vi "Longueur d'onde.vi"(11 "T thermistances":dbl[](array[numeric])) -> (3 "Wavelenght":dbl format="%#_13g")   [LabVIEW 2018]
uses:
  <vilib>/Analysis/baseanly.llb/Mean (DBL).vi
  <vilib>/Analysis/NI_AALBase.lvlib
  <vilib>/gmath/NI_Gmath.lvlib
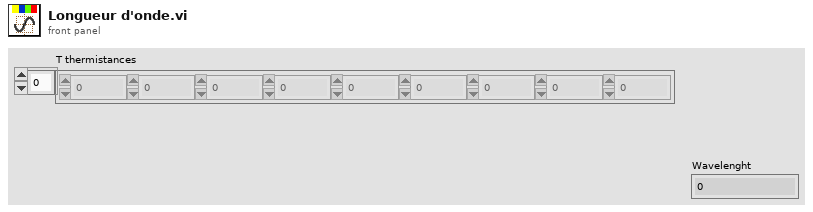
[diagram p1: front panel]
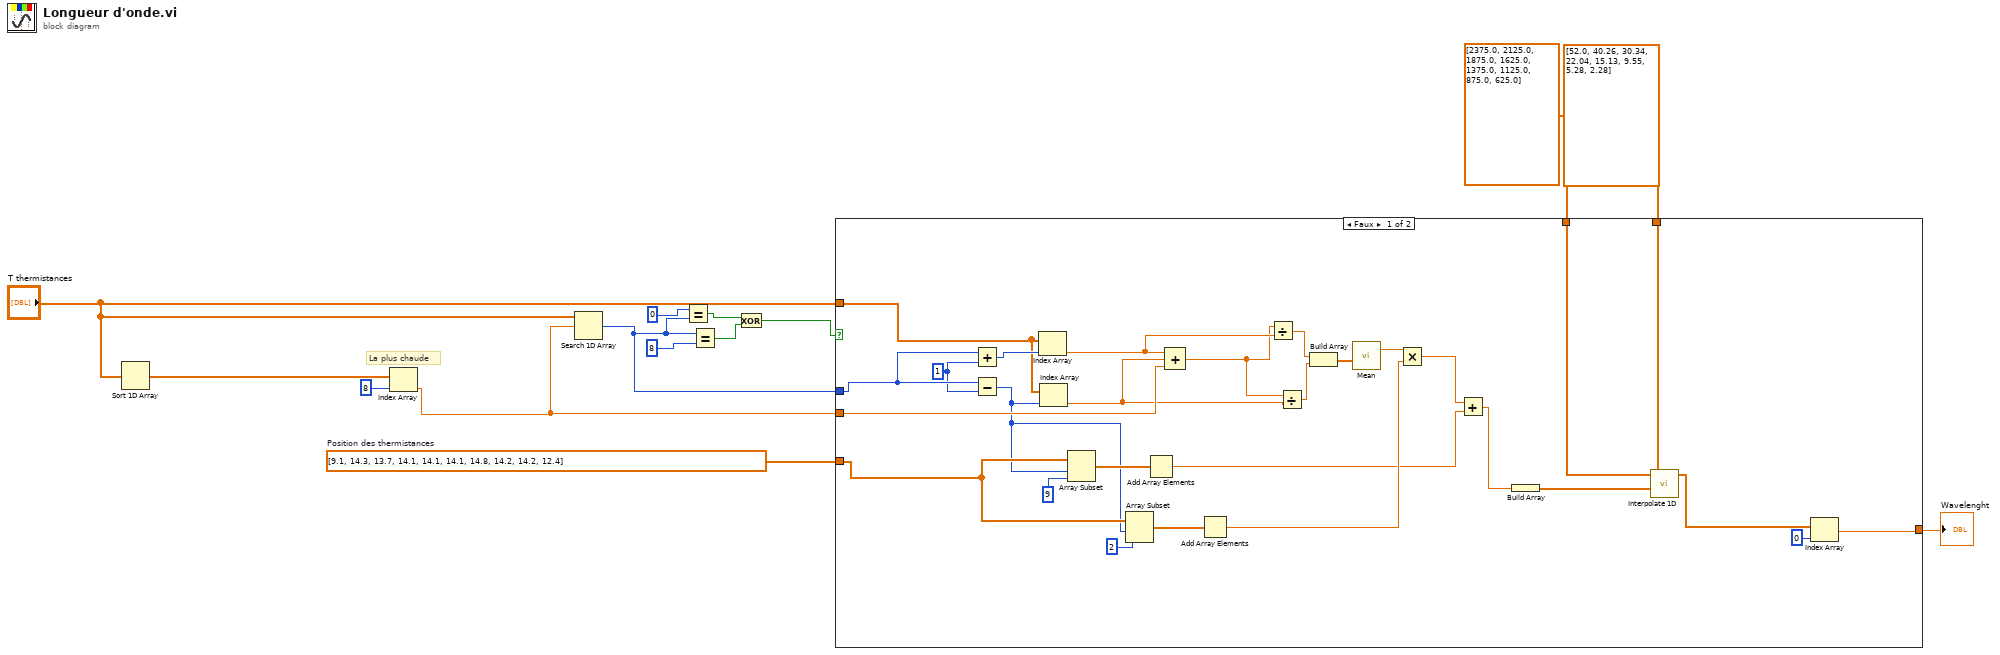
[diagram p0: block diagram]
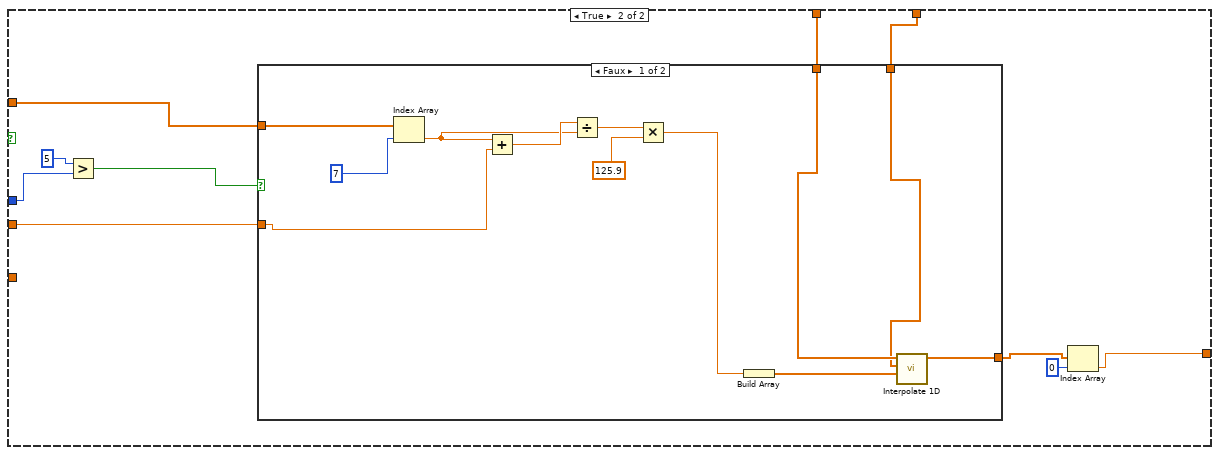
[diagram p2: hidden frame]
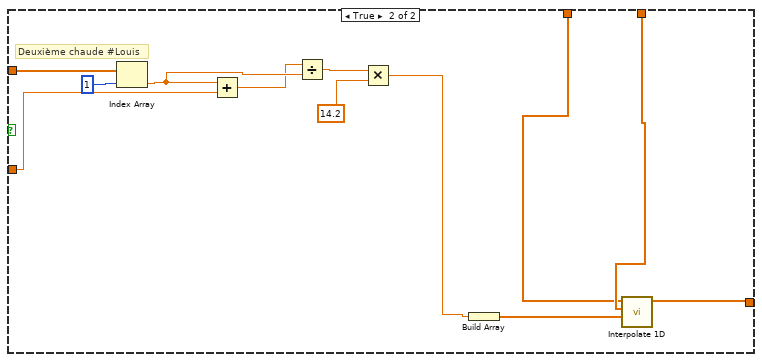
[diagram p3: hidden frame]
diagram:
  w4 = dbl[] [9.1, 14.3, 13.7, 14.1, 14.1, 14.1, 14.8, 14.2, 14.2, 12.4]  # Position des thermistances
  # "La plus chaude"
  n1 = Sort 1D Array(array="T thermistances") -> (sorted array=w13:dbl[])
  n2 = Index Array(array=w13, index=8 ("indice")) -> (element=w5:dbl)
  n3 = Search 1D Array(1D array="T thermistances", element=w5) -> (index of element=w10:i32)  [unwired: 1 in]
  n4 = Equal?(x=0, y=w10) -> (x = y?=w9:bool)
  n5 = Equal?(x=w10, y=8) -> (x = y?=w8:bool)
  n6 = Exclusive Or(1:w8, 2:w9) -> (0:w7:bool)
  n7 = case shown="Faux" w7 {
    tunnel: w10 -> [w42 w52]
    tunnel: "T thermistances" -> [w40 w49]
    tunnel: w5 -> [w38 w48]
    tunnel: w4 -> [w31 _]
    tunnel: [w18 w45] -> w3
    tunnel: dbl[] [52.0, 40.26, 30.34, 22.04, 15.13, 9.55, 5.28, 2.28] -> [w17 w43]
    tunnel: dbl[] [2375.0, 2125.0, 1875.0, 1625.0, 1375.0, 1125.0, 875.0, 625.0] -> [w16 w44]
    frame False {
      w39 = 1
      n8 = Add(x=w42, y=w39) -> (x+y=w41:i32)
      n9 = Subtract(x=w42, y=w39) -> (x-y=w29:i32)
      n10 = Index Array(array=w40, index=w41) -> (element=w23:dbl)
      n11 = Index Array(array=w40, index=w29) -> (element=w21:dbl)
      n12 = Array Subset(array=w31, index=w29, length=9) -> (w32:dbl[])
      n13 = Array Subset(array=w31, index=w29, length=2 ("longueur")) -> (w28:dbl[])
      n14 = Add Array Elements(numeric array=w32) -> (sum=w26:dbl)
      n15 = Compound Arithmetic op=ADD(w23, w21, w38) -> (w22:dbl)
      n16 = Add Array Elements(numeric array=w28) -> (sum=w27:dbl)
      n17 = Divide(x=w22, y=w23) -> (x/y=w36:dbl)
      n18 = Divide(x=w22, y=w21) -> (x/y=w37:dbl)
      n19 = Build Array(w36, w37) -> (w35:dbl[])
      n20 = call-poly <vilib>:"Mean.vi"("X"=w35) -> ("mean"=w33:dbl)  [unwired: 1 out]
      n21 = Multiply(x=w33, y=w27) -> (x*y=w25:dbl)
      n22 = Add(x=w25, y=w26) -> (x+y=w15:dbl)
      n23 = Build Array(w15) -> (w24:dbl[])
      n24 = call <vilib>:"Interpolate 1D.vi"("xi"=w24, "X"=w17, "Y"=w16) -> ("yi"=w20:dbl[])  [unwired: 6 in, 2 out]
      n25 = Index Array(array=w20, index=0 ("indice")) -> (element=w18:dbl)
    }
    frame True {
      n26 = Greater?(x=5, y=w52) -> (0:w50:bool)
      n27 = case shown="Faux" w50 {
        tunnel: w49 -> [w63 w76]
        tunnel: w48 -> [w56 w75]
        tunnel: [w55 w67] -> w46
        tunnel: w44 -> [w54 w65]
        tunnel: w43 -> [w53 w66]
        frame False {
          n28 = Index Array(array=w63, index=7) -> (element=w57:dbl)
          n29 = Add(x=w57, y=w56) -> (x+y=w62:dbl)
          n30 = Divide(x=w62, y=w57) -> (x/y=w60:dbl)
          n31 = Multiply(x=w60, y=125.9) -> (x*y=w58:dbl)
          n32 = Build Array(w58) -> (w59:dbl[])
          n33 = call <vilib>:"Interpolate 1D.vi"("xi"=w59, "X"=w53, "Y"=w54) -> ("yi"=w55:dbl[])  [unwired: 6 in, 2 out]
        }
        frame True {
          # "Deuxième chaude #Louis"
          n34 = Index Array(array=w76, index=1) -> (element=w73:dbl)
          n35 = Add(x=w73, y=w75) -> (x+y=w72:dbl)
          n36 = Divide(x=w72, y=w73) -> (x/y=w70:dbl)
          n37 = Multiply(x=w70, y=14.2) -> (x*y=w68:dbl)
          n38 = Build Array(w68) -> (w69:dbl[])
          n39 = call <vilib>:"Interpolate 1D.vi"("xi"=w69, "X"=w66, "Y"=w65) -> ("yi"=w67:dbl[])  [unwired: 6 in, 2 out]
        }
      }
      n40 = Index Array(array=w46, index=0 ("indice")) -> (element=w45:dbl)
    }
  }
  "Wavelenght" <- w3
